vi "BG Trim Bit - Write.vi"(8 "error in (no error)":errorcluster, 10 "BG Trim Bit":dbl[](array[numeric]), 11 "Globals in":refnum<class "TSM Context Data Access.lvclass">) -> (0 "error out":errorcluster, 3 "Globals out":refnum<class "TSM Context Data Access.lvclass">)   [LabVIEW 2019, in "TSM Context Data Access.lvclass"]
uses:
  TSM Context Data Access.lvclass
  TSM Context Data Access.lvclass/TSM Context Data Access.ctl
  <vilib>/NI_TestStand_SemiconductorModule/NI_TestStand_Semiconductor_Module.lvlibp
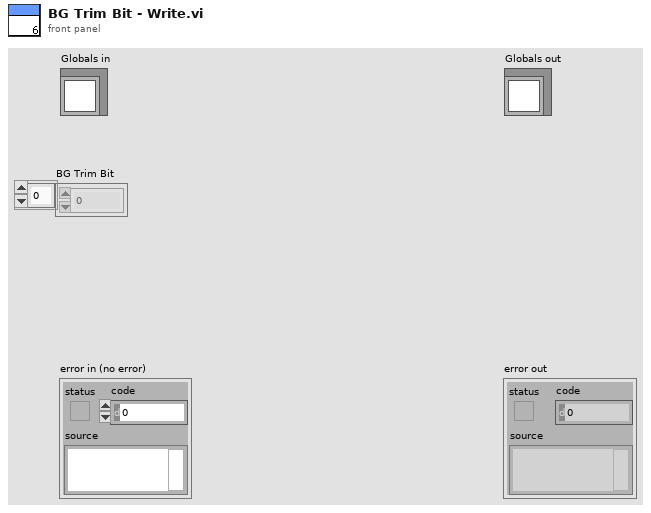
[diagram p1: front panel]
types:
  T1 = typedef "NI_TestStand_Semiconductor_Module.lvlibp/SemiconductorModuleContext.ctl" = refnum<k7>
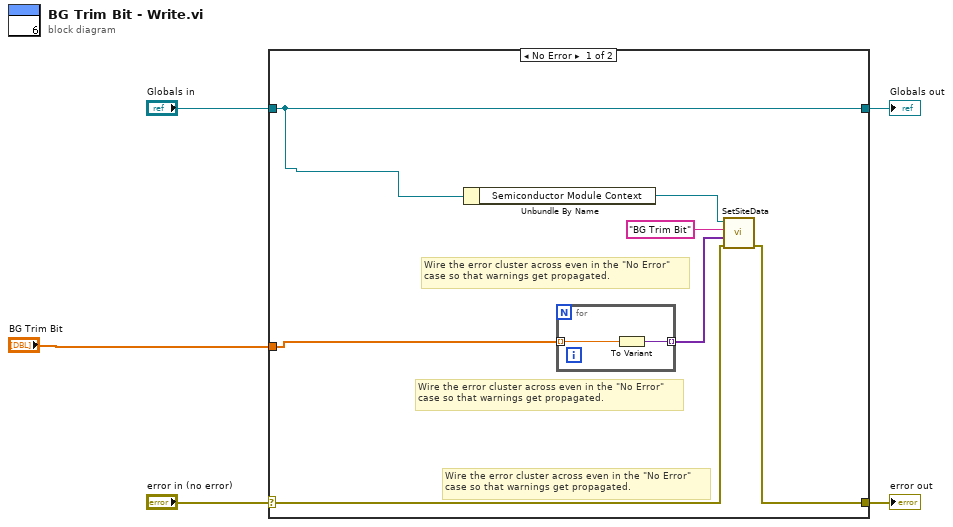
[diagram p0: block diagram]
diagram:
  n1 = case shown="No Error" "error in (no error)" {
    selector: "error in (no error)" -> [w8 w16]
    tunnel: [w7 w16] -> w4
    tunnel: [w9 w15] -> w2
    tunnel: "Globals in" -> [w9 w15]
    tunnel: "BG Trim Bit" -> [w6 _]
    frame No Error {
      # "Wire the error cluster across even in the \"No Error\"\ncase so that warnings get propagated."
      # "Wire the error cluster across even in the \"No Error\"\ncase so that warnings get propagated."
      # "Wire the error cluster across even in the \"No Error\"\ncase so that warnings get propagated."
      n2 = Unbundle By Name(w9) -> ("Semiconductor Module Context"=w12:T1)
      n3 = for {
        tunnel: [w14] -> w10 mode=indexing
        tunnel: w6 -> [w13] mode=indexing
        n4 = To Variant(anything=w13) -> (Variant=w14:variant)
      }
      n5 = call <vilib>:"SetSiteData.vi"("error in (no error)"=w8, "Site Data"=w10, "Data Id"="BG Trim Bit", "Semiconductor Module Context"=w12) -> ("error out"=w7:errorcluster)  [unwired: 5 in, 1 out]
    }
    frame Error {
    }
  }
  "error out" <- w4
  "Globals out" <- w2
